vi "HEAD.vi"(6 "timeout":i32=10000, 8 "error in":errorcluster, 10 "url":string, 11 "http-client in":refnum<class "http-client.lvclass">) -> (0 "error out":errorcluster, 2 "headers":string, 3 "http-client out":refnum<class "http-client.lvclass">)   [LabVIEW 2020, in "REST Client.lvlib" / "http-client.lvclass"]
uses:
  http-client.lvclass
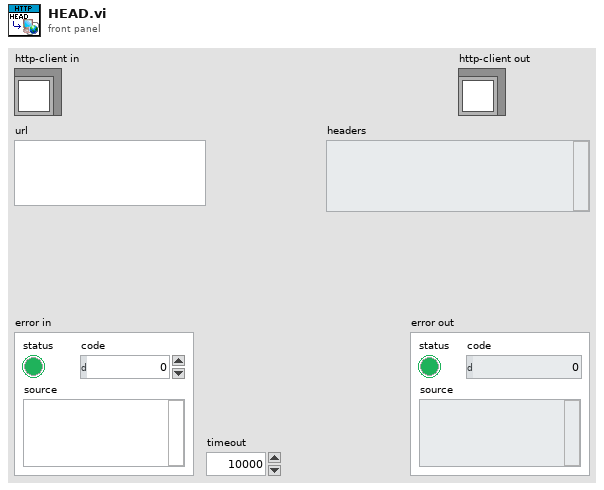
[diagram p1: front panel]
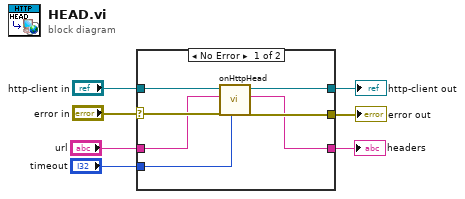
[diagram p0: block diagram]
diagram:
  n1 = case shown="No Error" "error in" {
    selector: "error in" -> [w12 w16]
    tunnel: [w11 w16] -> w6
    tunnel: [w14 w15] -> w4
    tunnel: "http-client in" -> [w13 w15]
    tunnel: [w10 _] -> w3
    tunnel: "url" -> [w9 _]
    tunnel: "timeout" -> [w8 _]
    frame No Error {
      n2 = call-dynamic "onHttpHead.vi"("timeout"=w8, "error in"=w12, "url"=w9, "http-method in"=w13) -> ("error out"=w11:errorcluster, "headers"=w10:string, "http-method out"=w14:refnum<class "http-client.lvclass">)  [unwired: 5 in]
    }
    frame Error {
    }
  }
  "error out" <- w6
  "http-client out" <- w4
  "headers" <- w3
